vi "DeCoF write characters.vi"(4 "error in (no error)":errorcluster, 6 "data in":string, 7 "Connection ID in":T1) -> (0 "error out":errorcluster, 3 "Conncection ID out":T1)   [LabVIEW 2013]
doc: "Writes any characters to the remote device."
uses:
  DeCoF connection.ctl
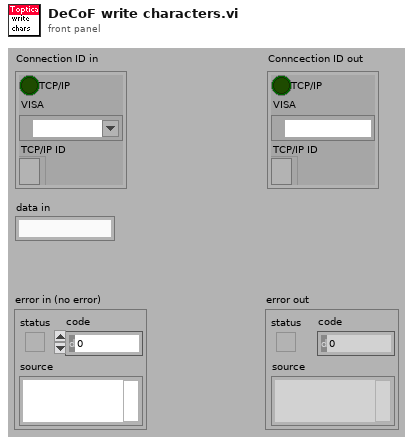
[diagram p1: front panel]
types:
  T1 = typedef "DeCoF connection.ctl" = cluster{"TCP/IP":bool, "VISA":refnum<visa-resource-name>, "TCP/IP ID":refnum<k5>}
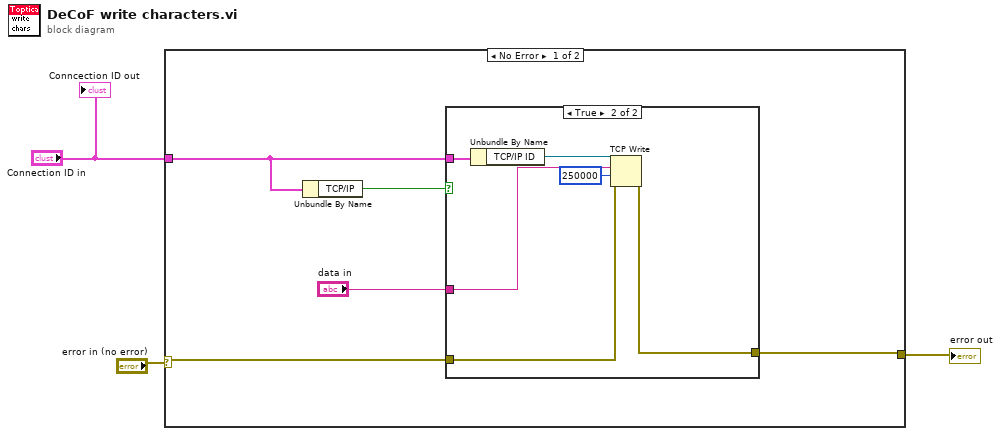
[diagram p0: block diagram]
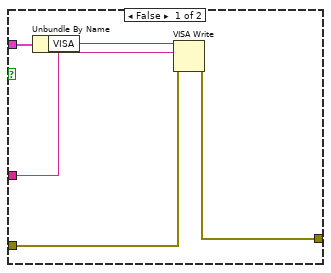
[diagram p2: hidden frame]
diagram:
  n1 = case shown="No Error" "error in (no error)" {
    selector: "error in (no error)" -> [w8 w20]
    tunnel: [w7 w20] -> w2
    tunnel: "Connection ID in" -> [w5 _]
    frame No Error {
      n2 = Unbundle By Name(w5) -> ("TCP/IP"=w4:bool)
      n3 = case shown="True" w4 {
        tunnel: w5 -> [w10 w16]
        tunnel: w8 -> [w13 w19]
        tunnel: [w12 w18] -> w7
        tunnel: "data in" -> [w11 w17]
        frame False {
          n4 = Unbundle By Name(w10) -> ("VISA"=w9:refnum<visa-resource-name>)
          n5 = VISA Write(VISA resource name=w9, write buffer=w11, error in (no error)=w13) -> (error out=w12:errorcluster)  [unwired: 2 out]
        }
        frame True {
          n6 = Unbundle By Name(w16) -> ("TCP/IP ID"=w15:refnum<k5>)
          n7 = TCP Write(connection ID=w15, data in=w17, error in (no error)=w19, 9:250000 ("timeout ms (25000)")) -> (error out=w18:errorcluster)  [unwired: 2 out]
        }
      }
    }
    frame Error {
    }
  }
  "error out" <- w2
  "Conncection ID out" <- "Connection ID in"
